vi "test.vi"() -> ()   [LabVIEW 2012, in "PassBouy.lvclass"]
uses:
  PassBouy.lvclass
  Data/TypeDefs/UTM Location.ctl
  Waypoint/Waypoint.lvclass
panel:
  in  "Y coord":dbl
  in  "X coord":dbl
  out "Waypoint Out":refnum<class "Waypoint.lvclass">
  in  "Points of Interest":T1[](array[typedef]) {"North" format="%#_10f"; "East" format="%#_8f"}
  in  "Base Point":enum16{"Port", "Midpoint", "Starboard"}(ring)
  in  "PassBouy.lvclass":refnum<class "PassBouy.lvclass">
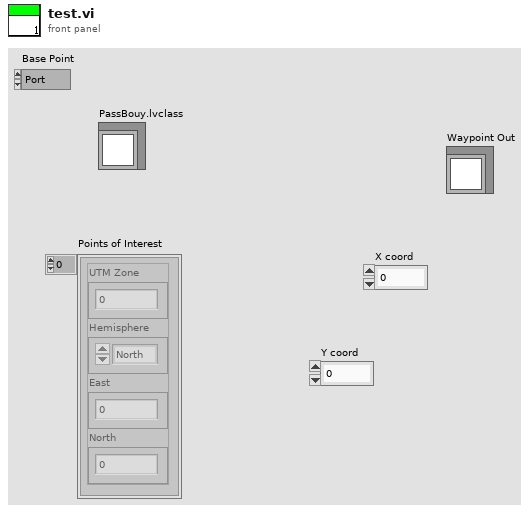
[diagram p1: front panel]
types:
  T1 = typedef "UTM Location.ctl" = cluster{"UTM Zone":dbl, "Hemisphere":enum16{"North", "South"}, "East":dbl, "North":dbl}
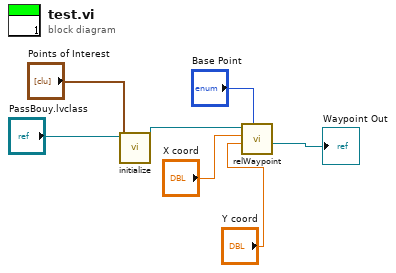
[diagram p0: block diagram]
diagram:
  n1 = call-dynamic "initialize.vi"("Points of Interest"="Points of Interest", "PassBouy.lvclass"="PassBouy.lvclass") -> ("PassBouy.lvclass out"=w5:refnum<class "PassBouy.lvclass">)  [unwired: 7 in, 1 out]
  n2 = call "relWaypoint.vi"("Base Point"="Base Point", "Y coord"="Y coord", "X coord"="X coord", "PassBouy.lvclass"=w5) -> ("Waypoint Out"=→"Waypoint Out":refnum<class "Waypoint.lvclass">)  [unwired: 5 in, 2 out]
